vi "MPU_Stick_Main_Init.vi"(8 "error in (no error)":errorcluster, 11 "MPU_Stick_Globals In":T1) -> (0 "error out":errorcluster, 3 "MPU_Stick_Globals Out":T1)   [LabVIEW 2017]
uses:
  Controls/MPU_Stick_Globals.ctl
  Controls/IMU_Configuration_References.ctl
  Controls/MP_Comp_Filter_Constants_References.ctl
  Controls/MD_Threshold_References.ctl
  Controls/MD_Type_References.ctl
  Controls/LED_Configuration_References.ctl
  Controls/Primary_References.ctl
  Controls/MPU_Stick_Queues.ctl
  Controls/MPU_Stick_Queue_Element.ctl
  Controls/MPU_Stick_Queue_Commands.ctl
  Classes/ADCP.lvclass
  Controls/MPU_Stick_Plotter_Core_Commands.ctl
  MPU_Stick_Read_Serial_Port_Emulator.vi
panel:
  in  "ADCP.lvclass":refnum<class "ADCP.lvclass">
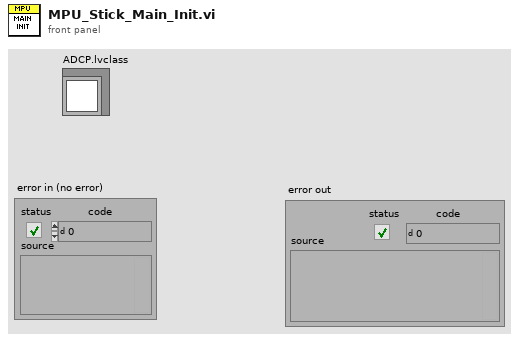
[diagram p1: front panel]
types:
  T1 = typedef "MPU_Stick_Globals.ctl" = cluster{"IMU_configuration_references":T2, "MP_Comp_Filter_Constants_References":T3, "MD_Threshold_References":T4, "MD_Type_References":T5, "LED_Configuration_References":T6, "Primary_references":T7, "MPU_Stick_Queues":T8, "ADCP":refnum<vi>}
  T2 = typedef "IMU_Configuration_References.ctl" = cluster{"Get all IMU configurations":refnum<vi>, "Set all IMU configurations":refnum<vi>, "Get sampling frequency":refnum<vi>, "Set sampling frequency":refnum<vi>, "Get calibration point count":refnum<vi>, "Set calibration point count":refnum<vi>, "Get calibration interval":refnum<vi>, "Set calibration interval":refnum<vi>, "Get Gyroscope bandwidth":refnum<vi>, "Set Gyroscope bandwidth":refnum<vi>, "Get Gyroscope F.S. Value":refnum<vi>, "Set Gyroscope F.S. Value":refnum<vi>, "Get Accelerometer bandwidth":refnum<vi>, "Set Accelerometer bandwidth":refnum<vi>, "Get Accelerometer F.S. Value":refnum<vi>, "Set Accelerometer F.S. Value":refnum<vi>, "Sampling frequency (Hz)":refnum<vi>, "Calibration point count":refnum<vi>, "Calibration interval (ms)":refnum<vi>, "IMU Gyroscope bandwidth":refnum<vi>, "IMU Gyroscope F.S. value":refnum<vi>, "IMU Accelerometer bandwidth":refnum<vi>, "IMU Accelerometer F.S. value":refnum<vi>}
  T3 = typedef "MP_Comp_Filter_Constants_References.ctl" = cluster{"Set pitch filter constant":refnum<vi>, "Get pitch filter constant":refnum<vi>, "Set roll filter constant":refnum<vi>, "Get roll filter constant":refnum<vi>, "Pitch filter constant":refnum<vi>, "Roll filter constant":refnum<vi>}
  T4 = typedef "MD_Threshold_References.ctl" = cluster{"Yaw threshold (U)":refnum<vi>, "Yaw threshold (L)":refnum<vi>, "Pitch threshold (U)":refnum<vi>, "Pitch. threshold (L)":refnum<vi>, "Roll threshold (U)":refnum<vi>, "Roll threshold (L)":refnum<vi>, "Z gyro. threshold (U)":refnum<vi>, "Z gyro. threshold (L)":refnum<vi>, "Y gyro. threshold (U)":refnum<vi>, "Y gyro. threshold (L)":refnum<vi>, "X gyro. threshold (U)":refnum<vi>, "X gyro. threshold (L)":refnum<vi>, "Z accel. threshold (U)":refnum<vi>, "Z accel. threshold (L)":refnum<vi>, "Y accel. threshold (U)":refnum<vi>, "Y accel. threshold (L)":refnum<vi>, "X accel. threshold (U)":refnum<vi>, "X accel. threshold (L)":refnum<vi>, "Set all Motion detection threshold configurations":refnum<vi>, "Get yaw threshold (upper)":refnum<vi>, "Get yaw threshold (lower)":refnum<vi>, "Get pitch threshold (upper)":refnum<vi>, "Get pitch threshold (lower)":refnum<vi>, "Get roll threshold (upper)":refnum<vi>, "Get roll threshold (lower)":refnum<vi>, "Get Z gyro threshold (upper)":refnum<vi>, "Get Z gyro threshold (lower)":refnum<vi>, "Get Y gyro threshold (upper)":refnum<vi>, "Get Y gyro threshold (lower)":refnum<vi>, "Get X gyro threshold (upper)":refnum<vi>, "Get X gyro threshold (lower)":refnum<vi>, "Get Z accel threshold (upper)":refnum<vi>, "Get Z accel threshold (lower)":refnum<vi>, "Get Y accel threshold (upper)":refnum<vi>, "Get Y accel threshold (lower)":refnum<vi>, "Get X accel threshold (upper)":refnum<vi>, "Get X accel threshold (lower)":refnum<vi>, "Get all Motion detection threshold configurations":refnum<vi>, "Set yaw threshold (upper)":refnum<vi>, "Set yaw threshold (lower)":refnum<vi>, "Set pitch threshold (upper)":refnum<vi>, "Set pitch threshold (lower)":refnum<vi>, "Set roll threshold (upper)":refnum<vi>, "Set roll threshold (lower)":refnum<vi>, "Set Z gyro threshold (upper)":refnum<vi>, "Set Z gyro threshold (lower)":refnum<vi>, "Set Y gyro threshold (upper)":refnum<vi>, "Set Y gyro threshold (lower)":refnum<vi>, "Set X gyro threshold (upper)":refnum<vi>, "Set X gyro threshold (lower)":refnum<vi>, "Set Z accel threshold (upper)":refnum<vi>, "Set Z accel threshold (lower)":refnum<vi>, "Set Y accel threshold (upper)":refnum<vi>, "Set Y accel threshold (lower)":refnum<vi>, "Set X accel threshold (upper)":refnum<vi>, "Set X accel threshold (lower)":refnum<vi>}
  T5 = typedef "MD_Type_References.ctl" = cluster{"Yaw threshold type":refnum<vi>, "Pitch threshold type":refnum<vi>, "Roll threshold type":refnum<vi>, "Z gyro threshold type":refnum<vi>, "Y gyro threshold type":refnum<vi>, "X gyro threshold type":refnum<vi>, "Z accel threshold type":refnum<vi>, "Y accel threshold type":refnum<vi>, "X accel threshold type":refnum<vi>, "Set all Motion detection type configurations":refnum<vi>, "Get all Motion detection type configurations":refnum<vi>, "Set yaw threshold type":refnum<vi>, "Get yaw threshold type":refnum<vi>, "Set pitch threshold type":refnum<vi>, "Get pitch threshold type":refnum<vi>, "Set roll threshold type":refnum<vi>, "Get roll threshold type":refnum<vi>, "Set Z gyroscope threshold type":refnum<vi>, "Get Z gyroscope threshold type":refnum<vi>, "Set Y gyroscope threshold type":refnum<vi>, "Get Y gyroscope threshold type":refnum<vi>, "Set X gyroscope threshold type":refnum<vi>, "Get X gyroscope threshold type":refnum<vi>, "Set Z accel threshold type":refnum<vi>, "Get Z accel threshold type":refnum<vi>, "Set Y accel threshold type":refnum<vi>, "Get Y accel threshold type":refnum<vi>, "Get X accel threshold type":refnum<vi>, "Set X accel threshold type":refnum<vi>}
  T6 = typedef "LED_Configuration_References.ctl" = cluster{"Get all LED configurations":refnum<vi>, "Set all LED configurations":refnum<vi>, "Get LED3 configuration":refnum<vi>, "Set LED3 configuration":refnum<vi>, "Get LED2 configuration":refnum<vi>, "Set LED2 configuration":refnum<vi>, "Get LED1 configuration":refnum<vi>, "Set LED1 configuration":refnum<vi>, "LED3 Configuration":refnum<vi>, "LED2 Configuration":refnum<vi>, "LED1 Configuration":refnum<vi>}
  T7 = typedef "Primary_References.ctl" = cluster{"3D View Image":refnum<vi>, "Plot":refnum<vi>, "Graph / 3D view tab control":refnum<vi>, "MP Reset":refnum<vi>, "Calibrate IMU":refnum<vi>, "Plot Parameter List":refnum<vi>, "Remove Parameter from Plot":refnum<vi>, "Add Parameter to Plot":refnum<vi>, "Parameter to monitor":refnum<vi>, "Yaw motion detection output":refnum<vi>, "Pitch motion detection output":refnum<vi>, "Roll motion detection output":refnum<vi>, "Z gyro motion detection output":refnum<vi>, "Y gyro motion detection output":refnum<vi>, "X gyro motion detection output":refnum<vi>, "Z accel motion detection output":refnum<vi>, "Y accel motion detection output":refnum<vi>, "X accel motion detection output":refnum<vi>, "Yaw angle (filter) (degrees)":refnum<vi>, "Pitch angle (filter) (degrees)":refnum<vi>, "Roll angle (filter) (degrees)":refnum<vi>, "Yaw angle (gyro) (degrees)":refnum<vi>, "Pitch angle (gyro) (degrees)":refnum<vi>, "Roll angle (gyro) (degrees)":refnum<vi>, "Yaw angle (accel) (degrees)":refnum<vi>, "Pitch angle (accel) (degrees)":refnum<vi>, "Roll angle (accel) (degrees)":refnum<vi>, "Z gyroscope reading (DPS)":refnum<vi>, "Y gyroscope reading (DPS)":refnum<vi>, "X gyroscope reading (DPS)":refnum<vi>, "Z accelerometer reading (G)":refnum<vi>, "Y accelerometer reading (G)":refnum<vi>, "X accelerometer reading (G)":refnum<vi>, "Save all config.":refnum<vi>, "Write all config.":refnum<vi>, "Read all config.":refnum<vi>, "Tab Control":refnum<vi>, "Baud Rate":refnum<vi>, "COM Port":refnum<vi>, "Time (ms)":refnum<vi>, "Value (Units)":refnum<vi>, "Exit Application":refnum<vi>, "Connect Device":refnum<vi>, "Progress Bar":refnum<vi>, "Get Range & Offset":refnum<vi>, "Range":refnum<vi>, "Offset":refnum<vi>, "Set Range & Offset":refnum<vi>, "Parameter name":refnum<vi>, "Plot time (ms)":refnum<vi>, "Plot value":refnum<vi>}
  T8 = typedef "MPU_Stick_Queues.ctl" = cluster{"UI Event Handler":refnum<queue>, "3D View Updater":refnum<queue>, "Plot Updater":refnum<queue>, "Serial Port Reader":refnum<queue>, "UI Indicators Updater":refnum<queue>}
  T9 = typedef "MPU_Stick_Plotter_Core_Commands.ctl" = enum16{"Initialize", "Add Channel", "Remove Channel", "Set Channel Minimum Value", "Set Channel Maximum Value", "Set Offset & Multiplier", "Get Offset & Multiplier", "Update Channel", "Get Cursor Data", "Clear", "Reset"}
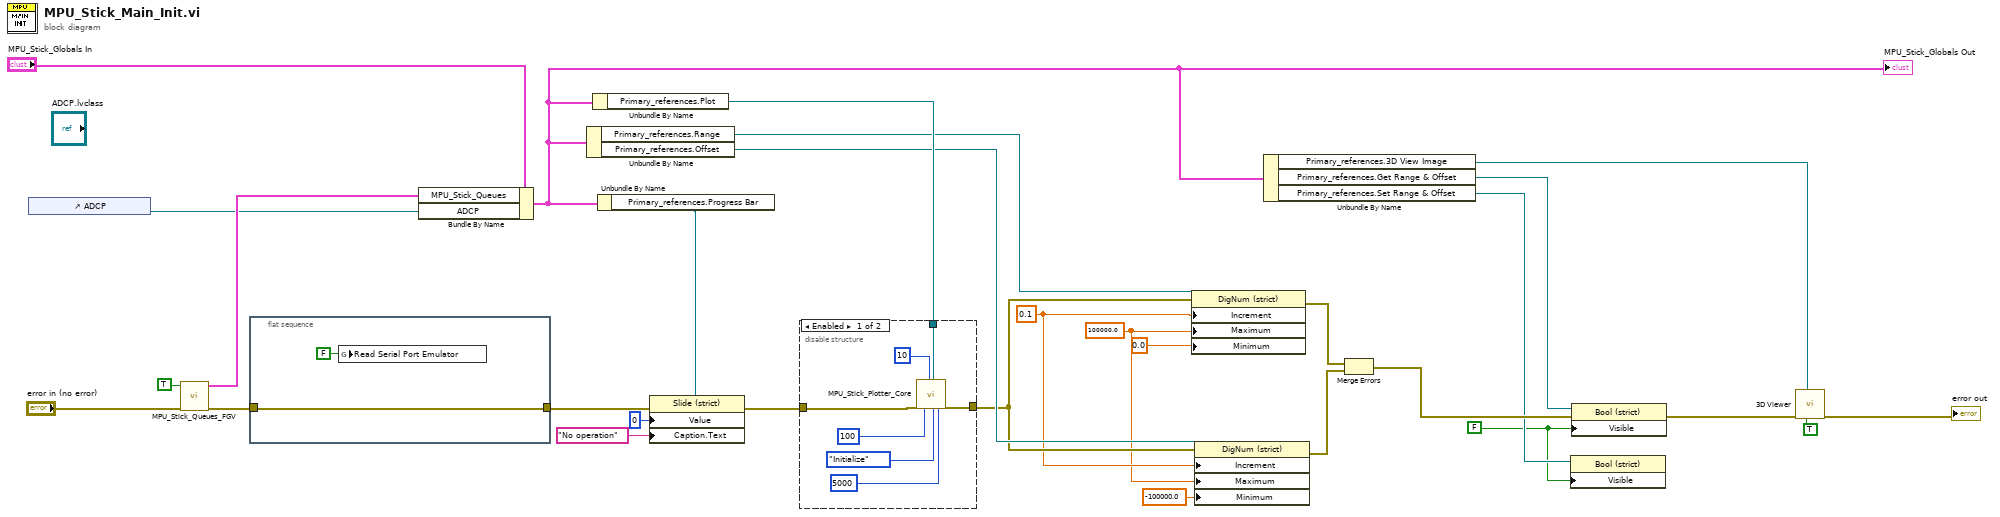
[diagram p0: block diagram]
diagram:
  w7 = FALSE ("Visible")
  w14 = 100000.0 ("Data Entry Limits:Maximum")
  w15 = 0.1 ("Data Entry Limits:Increment")
  n1 = control-ref of="ADCP"() -> (w26:refnum<vi>)
  n2 = call "MPU_Stick_Queues_FGV.vi"("error in (no error)"="error in (no error)", "Initialize ?"=TRUE) -> ("error out"=w2:errorcluster, "MPU_Stick_Queues"=w27:T8)  [unwired: 8 in]
  n3 = flat-sequence {
    tunnel: w2 -> [w31]
    tunnel: [w31] -> w1
    frame #0 {
      n4 = global write "MPU_Stick_Read_Serial_Port_Emulator.vi" "Read Serial Port Emulator"(FALSE ("Read Serial Port Emulator")) -> ()
    }
  }
  n5 = Bundle By Name(cluster="MPU_Stick_Globals In", "MPU_Stick_Queues"=w27, "ADCP"=w26) -> (w11:T1)
  "MPU_Stick_Globals Out" <- w11
  n6 = Unbundle By Name(w11) -> ("Primary_references.Range"=w20:refnum<vi>, "Primary_references.Offset"=w19:refnum<vi>)
  n7 = Unbundle By Name(w11) -> ("Primary_references.Plot"=w21:refnum<vi>)
  n8 = Unbundle By Name(w11) -> ("Primary_references.Progress Bar"=w25:refnum<vi>)
  n9 = property class="Slide (strict)"(reference=w25, error in=w1, "Value"=u8 0, "Caption.Text"="No operation" ("Label.Text")) -> (error out=w22:errorcluster)  [unwired: 1 out]
  n10 = disable-structure shown="Enabled" {
    disable-tunnel: w22 -> [w39 w40]
    disable-tunnel: w21 -> [w38 _]
    disable-tunnel: [w34 w40] -> w18
    frame Enabled {
      n11 = call "MPU_Stick_Plotter_Core.vi"("error in (no error)"=w39, "Plot update interval (ms)"=u32 100, "Number of vertical divisions"=u16 10, "Plot reference"=w38, "Command"=MPU_Stick_Plotter_Core_Commands."Initialize", "Time axis length (ms)"=u32 5000) -> ("error out"=w34:errorcluster)  [unwired: 10 in, 3 out]
    }
    frame Disabled {
    }
  }
  n12 = property class="DigNum (strict)"(reference=w20, error in=w18, "Increment"=w15, "Maximum"=w14, "Minimum"=0.0 ("Data Entry Limits:Minimum")) -> (error out=w17:errorcluster)  [unwired: 1 out]
  n13 = property class="DigNum (strict)"(reference=w19, error in=w18, "Increment"=w15, "Maximum"=w14, "Minimum"=-100000.0 ("Data Entry Limits:Minimum")) -> (error out=w16:errorcluster)  [unwired: 1 out]
  n14 = Unbundle By Name(w11) -> ("Primary_references.3D View Image"=w3:refnum<vi>, "Primary_references.Get Range & Offset"=w9:refnum<vi>, "Primary_references.Set Range & Offset"=w8:refnum<vi>)
  n15 = Merge Errors(w17, w16) -> (w10:errorcluster)
  n16 = property class="Bool (strict)"(reference=w8, "Visible"=w7) -> ()  [unwired: 1 in, 2 out]
  n17 = property class="Bool (strict)"(reference=w9, error in=w10, "Visible"=w7) -> (error out=w6:errorcluster)  [unwired: 1 out]
  n18 = call "3D Viewer.vi"("Initialize ?"=TRUE, "3D View Image"=w3, "error in (no error)"=w6) -> ("error out"=→"error out":errorcluster)  [unwired: 7 in, 1 out]
